vi "Main.vi"() -> ()   [LabVIEW 2021]
uses:
  <vilib>/FPGAPlugInAG/myRIO-1900/niLvFpga_Open_myRIO-1900.vi
  <vilib>/rvi/interface/common/dynamic/niFpgaDynamicAddResources.vi
  <vilib>/addons/Time Frequency Analysis/Spectrogram.llb/TFA Online STFT Spectrogram (Waveform).vi
  <vilib>/addons/Time Frequency Analysis/_control.llb/TFA Configure Spectrogram Indicator (Predefined Color Table).vi
  <vilib>/FPGAPlugInAG/Dynamic/niLvFpga_Close_Dynamic.vi
  <vilib>/rvi/interface/nirviOpenFPGA/nirviOpenFPGA.xnode
  FPGA Bitfiles/FPGA Audio Streaming (with LEDs).lvbitx
  FPGA Audio Streaming.vi
  <vilib>/rvi/interface/nirviCloseFPGA/nirviCloseFPGA.xnode
  <vilib>/addons/_Advanced Signal Processing/NI_AdvSigProcTFA.lvlib
panel:
  in  "Window Information":cluster{"Type":i32, "Length":i32}={"Type"=1, "Length"=512} {"Type" items=["None ", "Hanning", "Hamming", "Blackman-Harris", "Exact Blackman", "Blackman", "Flat Top"]}
  out "Raw Audio Signal":i16[](graph)
  out "Real-Time Spectrogram":dbl[][](graph)
  in  "stop":bool
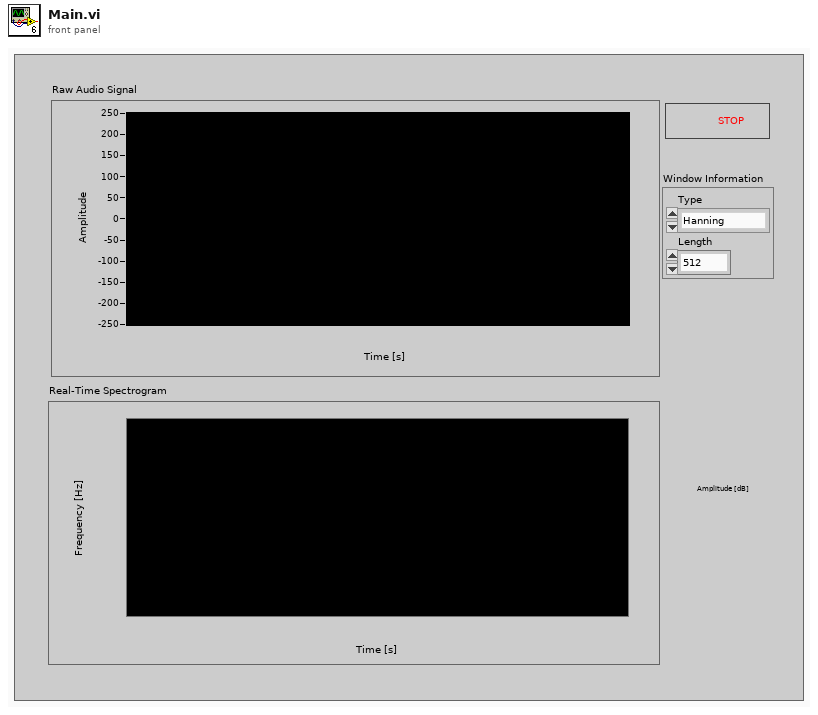
[diagram p1: front panel]
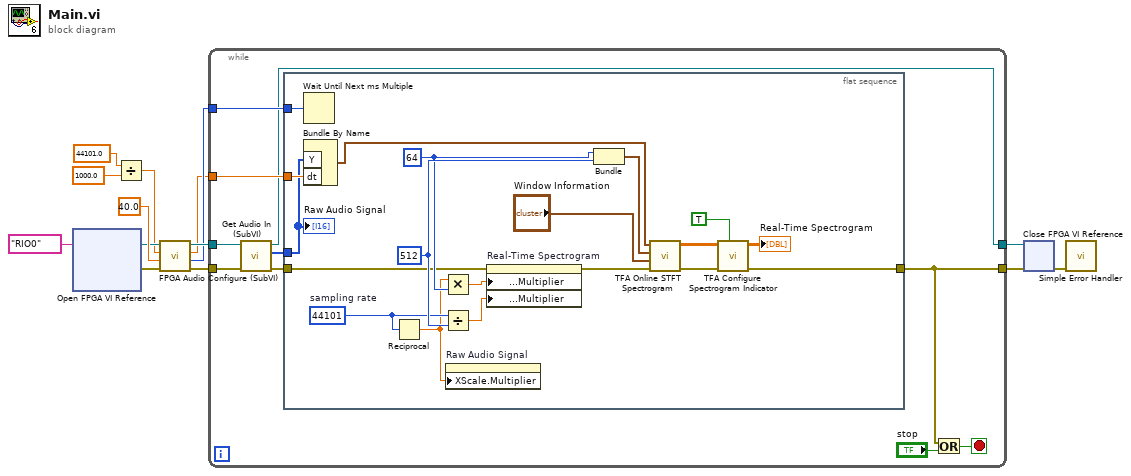
[diagram p0: block diagram]
diagram:
  n1 = xnode "Open FPGA VI Reference"("resource name"=tag "RIO0") -> ("FPGA VI Reference Out"=w7:refnum<k20>, "error out"=w14:errorcluster)  [unwired: 1 in]
  n2 = Divide(x=44101.0 ("Sample Rate (kHz)"), y=1000.0) -> (x/y=w2:dbl)
  n3 = call "FPGA Audio Configure (SubVI).vi"("error in (no error)"=w14, "Read Rate (Hz)"=40.0, "Audio Sample Rate (kHz)"=w2, "Refnum in"=w7) -> ("error out"=w9:errorcluster, "Required loop period (ms)"=w6:u32, "Audio dt (ms)"=w4:dbl, "Refnum out"=w13:refnum<k20>)  [unwired: 4 in]
  n4 = while {
    tunnel: w13 -> [w21]
    tunnel: [w17] -> w12
    tunnel: [w15] -> w11
    tunnel: w6 -> [w18]
    tunnel: w9 -> [w22]
    tunnel: w4 -> [w20]
    stop <- w23 stop-if-true
    n5 = call "Get Audio In (SubVI).vi"("error in (no error)"=w22, "Refnum in"=w21) -> ("error out"=w16:errorcluster, "Left Audio In"=w19:i16[], "Refnum out"=w17:refnum<k20>)  [unwired: 6 in, 1 out]
    n6 = flat-sequence {
      tunnel: w20 -> [w32]
      tunnel: w19 -> [w27]
      tunnel: w18 -> [w29]
      tunnel: w16 -> [w31]
      tunnel: [w30] -> w15
      frame #0 {
        w40 = 44101  # sampling rate
        w43 = 512 ("Frequency bins")
        w41 = 64 ("Time steps")
        n7 = Wait Until Next ms Multiple(millisecond multiple=w29) -> ()  [unwired: 1 out]
        n8 = Bundle By Name("Y"=w27, "dt"=w32) -> (w28:waveform(i16))  [unwired: 1 in]
        n9 = Reciprocal(x=w40) -> (1/x=w26:dbl)
        n10 = Multiply(x=w26, y=w41) -> (x*y=w38:dbl)
        n11 = Divide(x=w40, y=w43) -> (x/y=w42:dbl)
        n12 = property on="Raw Audio Signal" class="WFChart (strict)"("XScale.Multiplier"=w26) -> ()  [unwired: 2 in, 2 out]
        n13 = property on="Real-Time Spectrogram" class="IntChart (strict)"(error in=w31, "X Scale.Offset and Multiplier:Multiplier"=w38, "Y Scale.Offset and Multiplier:Multiplier"=w42) -> (error out=w39:errorcluster)  [unwired: 1 in, 1 out]
        n14 = Bundle("Time steps"=w41, "Frequency bins"=w43) -> (w37:cluster{"Time steps":i32, "Frequency bins":i32})  [unwired: 1 out]
        n15 = call-poly <vilib>:"TFA Online STFT Spectrogram.vi"("error in (no error)"=w39, "window info"="Window Information", "time-frequency sampling info"=w37, "signal"=w28) -> ("error out"=w33:errorcluster, "spectrogram"=w36:dbl[][])  [unwired: 6 out]
        n16 = call-poly <vilib>:"TFA Configure Spectrogram Indicator.vi"("dB on? (F)"=TRUE ("dB? (F)"), "error in (no error)"=w33, "spectrogram"=w36) -> ("error out"=w30:errorcluster, "TF spectrogram indicator"=→"Real-Time Spectrogram":dbl[][])  [unwired: 4 in, 3 out]
        "Raw Audio Signal" <- w27
      }
    }
    n17 = Or(x=w15, y="stop") -> (x .or. y?=w23:bool)
  }
  n18 = xnode "Close FPGA VI Reference"("FPGA VI Reference In"=w12, "error in"=w11) -> ("error out"=w5:errorcluster)
  n19 = call <vilib>:"Simple Error Handler.vi"("error in (no error)"=w5) -> ()  [unwired: 4 in, 5 out]
